vi "IniFiles.vi"(8 "error in":errorcluster, 10 "iniKey":string="pluginType", 11 "name or relative path":string="MyPlugins") -> (0 "error out":errorcluster, 2 "Types":string[](array[string]), 3 "IniFilePaths":path[](array[path]))   [LabVIEW 2014, in "ScopeModule.lvlib"]
uses:
  ScopeModule.lvlib
  <vilib>/Utility/config.llb/Read Key (String).vi
  <vilib>/Utility/config.llb/NI_LVConfig.lvlib
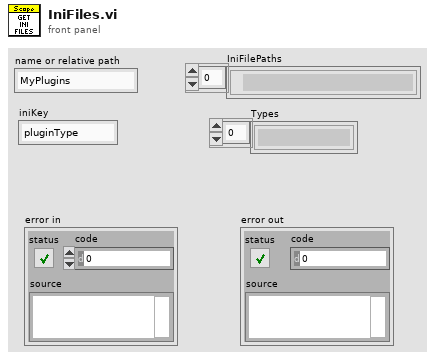
[diagram p1: front panel]
types:
  T1 = typedef "NI_LVConfig.lvlib/Config Data RefNum.ctl" = refnum<k1>
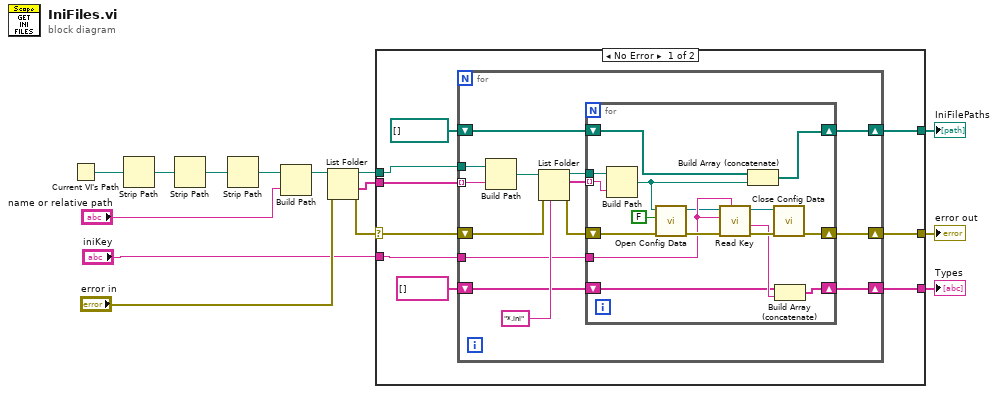
[diagram p0: block diagram]
diagram:
  n1 = Current VI's Path() -> (path=w14:path)
  n2 = Strip Path(path=w14) -> (stripped path=w13:path)  [unwired: 1 out]
  n3 = Strip Path(path=w13) -> (stripped path=w12:path)  [unwired: 1 out]
  n4 = Strip Path(path=w12) -> (stripped path=w11:path)  [unwired: 1 out]
  n5 = Build Path(base path=w11, name or relative path="name or relative path") -> (appended path=w9:path)
  n6 = List Folder(path=w9, error in="error in") -> (path out=w7:path, folder names=w6:string[], error out=w8:errorcluster)  [unwired: 2 in, 1 out]
  n7 = case shown="No Error" w8 {
    selector: w8 -> [w22 w54]
    tunnel: w7 -> [w21 _]
    tunnel: w6 -> [w23 _]
    tunnel: [w19 _] -> w5
    tunnel: [w18 w54] -> w3
    tunnel: "iniKey" -> [w17 _]
    tunnel: [w15 _] -> w1
    frame No Error {
      n8 = for {
        tunnel: w23 -> [w37] mode=indexing
        shift-right: [w24] -> w18
        shift-left: w22 -> [w35]
        tunnel: w21 -> [w36]
        shift-right: [w30] -> w19
        shift-left: path[] [] -> [w29]
        tunnel: w17 -> [w27]
        shift-right: [w26] -> w15
        shift-left: string[] [] -> [w25]
        n9 = Build Path(base path=w36, name or relative path=w37) -> (appended path=w33:path)
        n10 = List Folder(path=w33, pattern="*.ini", error in=w35) -> (path out=w31:path, filenames=w32:string[], error out=w28:errorcluster)  [unwired: 1 in, 1 out]
        n11 = for {
          tunnel: w32 -> [w52] mode=indexing
          tunnel: w31 -> [w53]
          shift-right: [w51] -> w30
          shift-left: w29 -> [w50]
          shift-right: [w42] -> w24
          shift-left: w28 -> [w47]
          tunnel: w27 -> [w45]
          shift-right: [w41] -> w26
          shift-left: w25 -> [w39]
          n12 = Build Path(base path=w53, name or relative path=w52) -> (appended path=w49:path)
          n13 = call <vilib>:"Open Config Data.vi"("error in (no error)"=w47, "create file if necessary (T)"=FALSE, "configuration file path"=w49) -> ("error out"=w46:errorcluster, "refnum"=w38:T1)  [unwired: 6 in, 1 out]
          n14 = call-poly <vilib>:"Read Key.vi"("section"=w45, "error in (no error)"=w46, "key"=w45, "refnum"=w38) -> ("error out"=w44:errorcluster, "value"=w40:string, "refnum out"=w43:T1)  [unwired: 4 in, 1 out]
          n15 = Build Array (concatenate)(w50, w49) -> (w51:path[])
          n16 = call <vilib>:"Close Config Data.vi"("error in (no error)"=w44, "refnum"=w43) -> ("error out"=w42:errorcluster)  [unwired: 8 in, 1 out]
          n17 = Build Array (concatenate)(w39, w40) -> (w41:string[])
        }
      }
    }
    frame Error {
    }
  }
  "IniFilePaths" <- w5
  "error out" <- w3
  "Types" <- w1
